vi "Pumping_Water.vi"(1 "Numeric 2":dbl) -> ()   [LabVIEW 2020]
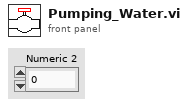
[diagram p1: front panel]
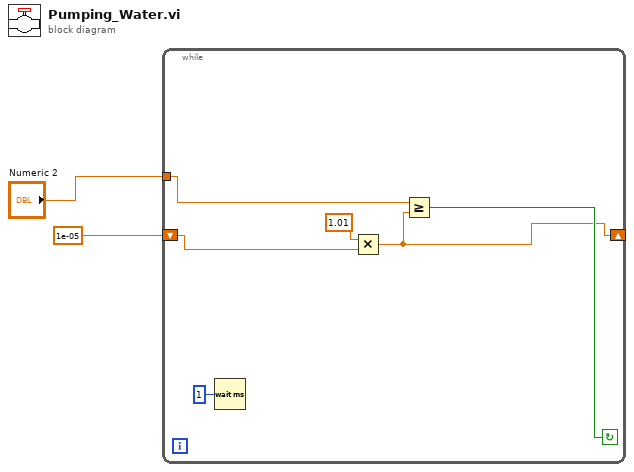
[diagram p0: block diagram]
diagram:
  n1 = while {
    tunnel: "Numeric 2" -> [w7]
    shift-right: [w3] -> _
    shift-left: 1e-05 -> [w4]
    stop <- w6 continue-if-true
    n2 = Wait (ms)(milliseconds to wait=u32 1) -> ()  [unwired: 1 out]
    n3 = Multiply(x=1.01, y=w4) -> (x*y=w3:dbl)
    n4 = Greater Or Equal?(x=w7, y=w3) -> (x >= y?=w6:bool)
  }
